vi "Acquire Class Reference.vi"(8 "error in (no error)":errorcluster, 11 "ParentClass in":refnum<class "ParentClass.lvclass">) -> (0 "error out":errorcluster, 2 "Class Reference":refnum<data-value>, 3 "ParentClass out":refnum<class "ParentClass.lvclass">)   [LabVIEW 2012, in "ParentClass.lvclass"]
uses:
  ParentClass.lvclass
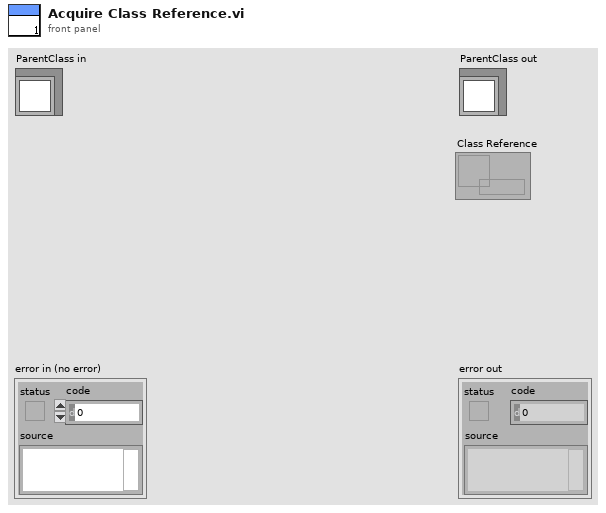
[diagram p1: front panel]
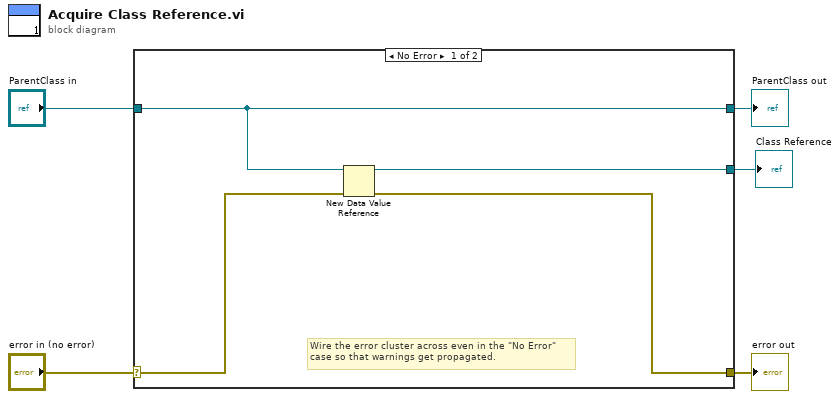
[diagram p0: block diagram]
diagram:
  n1 = case shown="No Error" "error in (no error)" {
    selector: "error in (no error)" -> [w8 w11]
    tunnel: [w7 w11] -> w4
    tunnel: [w9 w10] -> w2
    tunnel: "ParentClass in" -> [w9 w10]
    tunnel: [w6 _] -> w1
    frame No Error {
      # "Wire the error cluster across even in the \"No Error\"\ncase so that warnings get propagated."
      n2 = New Data Value Reference(data value=w9, error in=w8) -> (data value reference=w6:refnum<data-value>, error out=w7:errorcluster)
    }
    frame Error {
    }
  }
  "error out" <- w4
  "ParentClass out" <- w2
  "Class Reference" <- w1
